vi "SET_ActiveGlyph.vi"(8 "error in (no error)":errorcluster, 10 "Active Glyph":T1, 11 "Glyph in":refnum<class "Glyph.lvclass">) -> (0 "error out":errorcluster, 3 "Glyph out":refnum<class "Glyph.lvclass">)   [LabVIEW 2021, in "Glyph.lvclass"]
uses:
  <resource>/plugins/NIIconEditor/Class/Icon Library/Glyph.lvclass
  <vilib>/LabVIEW Icon API/lv_icon/Controls/Graphic.ctl
  <resource>/plugins/NIIconEditor/Class/Icon Library/Glyph.lvclass/Glyph.ctl
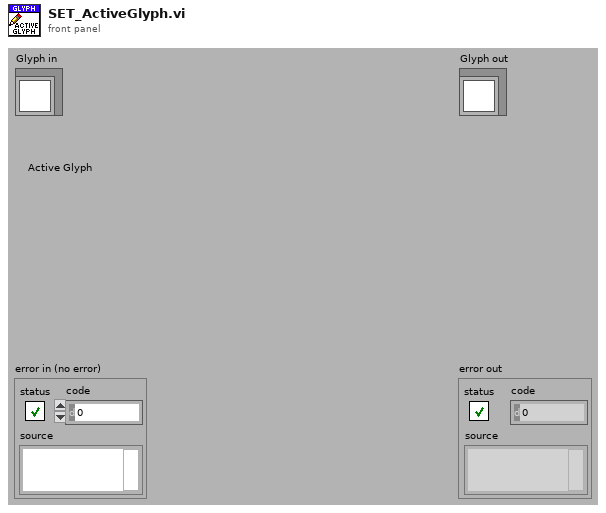
[diagram p1: front panel]
types:
  T1 = typedef "Graphic.ctl" = cluster{"Rectangle":cluster{"left":i16, "top":i16, "right":i16, "bottom":i16}, "Path":path, "Image":picture, "Filter":string, "FileName":string}
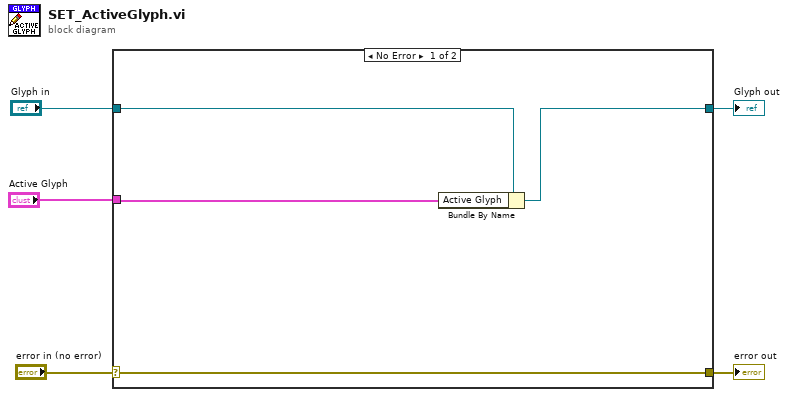
[diagram p0: block diagram]
diagram:
  n1 = case shown="No Error" "error in (no error)" {
    selector: "error in (no error)" -> [w9 w11]
    tunnel: [w9 w11] -> w4
    tunnel: [w7 w10] -> w2
    tunnel: "Glyph in" -> [w8 w10]
    tunnel: "Active Glyph" -> [w6 _]
    frame No Error {
      n2 = Bundle By Name(cluster=w8, "Active Glyph"=w6) -> (w7:refnum<class "Glyph.lvclass">)
    }
    frame Error {
    }
  }
  "error out" <- w4
  "Glyph out" <- w2
